vi "Heat2D_X Extend U(n).vi"(5 "Coefficients":T1={"rx"=0.0, "ry"=0.0, "s"=-0.0, "c"=0.0, "deltaT"=0.0, "deltaX"=0.0, "deltaY"=0.0}, 7 "step":i32, 10 "U(n)":dbl[][](array[numeric]), 11 "Boundary Condition":cluster{"type":T2, "Value":dbl[][]}[](array[cluster]) {"type" items=["Dirichlet", "Neumann"]}) -> (2 "Interp(X)":dbl[][](array[numeric]))   [LabVIEW 2017, in "NI_PDE.lvlib"]
uses:
  <vilib>/gmath/NI_PDE.lvlib
  <vilib>/gmath/pde.llb/Common/PDE_BC Type.ctl
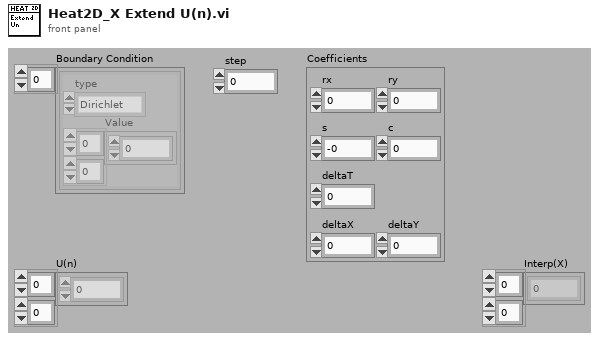
[diagram p1: front panel]
types:
  T1 = cluster{"rx":dbl, "ry":dbl, "s":dbl, "c":dbl, "deltaT":dbl, "deltaX":dbl, "deltaY":dbl}
  T2 = typedef "NI_PDE.lvlib/PDE_BC Type.ctl" = i32
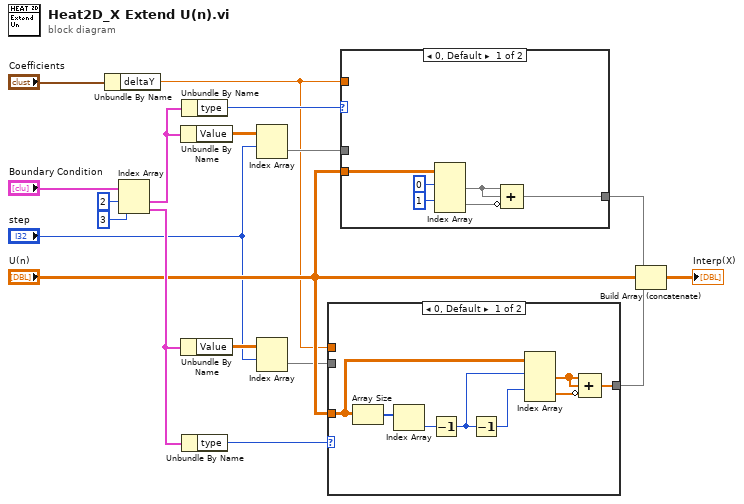
[diagram p0: block diagram]
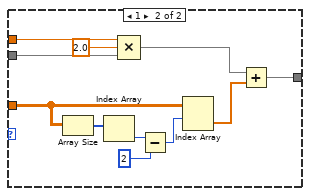
[diagram p2: hidden frame]
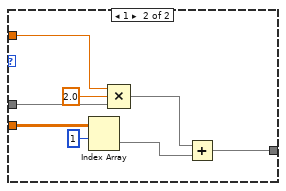
[diagram p3: hidden frame]
diagram:
  n1 = Unbundle By Name("Coefficients") -> ("deltaY"=w2:dbl)
  n2 = Index Array(array="Boundary Condition", index #1=2 ("index"), index #2=3 ("index")) -> (element #1=w11:cluster{"type":T2, "Value":dbl[][]}, element #2=w6:cluster{"type":T2, "Value":dbl[][]})
  n3 = Unbundle By Name(w11) -> ("Value"=w10:dbl[][])
  n4 = Unbundle By Name(w6) -> ("Value"=w5:dbl[][])
  n5 = Unbundle By Name(w11) -> ("type"=w12:T2)
  n6 = Unbundle By Name(w6) -> ("type"=w7:T2)
  n7 = Index Array(array=w10, index (row)="step") -> (element=w9:dbl[])  [unwired: 1 in]
  n8 = Index Array(array=w5, index (row)="step") -> (element=w3:dbl[])  [unwired: 1 in]
  n9 = case shown="0, Default" w7 {
    tunnel: [w26 w28] -> w17
    tunnel: "U(n)" -> [w19 w35]
    tunnel: w3 -> [_ w31]
    tunnel: w2 -> [_ w30]
    frame 0, Default {
      n10 = Array Size(array=w19) -> (size(s)=w25:i32[])
      n11 = Index Array(array=w25) -> (element=w24:i32)  [unwired: 1 in]
      n12 = Decrement(x=w24) -> (x-1=w20:i32)
      n13 = Decrement(x=w20) -> (x-1=w23:i32)
      n14 = Index Array(array=w19, index (row) #1=w20, index (row) #2=w23) -> (element #1=w22:dbl[], element #2=w21:dbl[])  [unwired: 2 in]
      n15 = Compound Arithmetic op=ADD(w22, w22, invert w21) -> (w26:dbl[])
    }
    frame 1 {
      n16 = Array Size(array=w35) -> (size(s)=w37:i32[])
      n17 = Index Array(array=w37) -> (element=w36:i32)  [unwired: 1 in]
      n18 = Compound Arithmetic op=MULTIPLY(w30, 2.0, w31) -> (w29:dbl[])
      n19 = Subtract(x=w36, y=2 ("index (row)")) -> (x-y=w33:i32)
      n20 = Index Array(array=w35, index (row)=w33) -> (element=w27:dbl[])  [unwired: 1 in]
      n21 = Add(x=w29, y=w27) -> (x+y=w28:dbl[])
    }
  }
  n22 = case shown="0, Default" w12 {
    tunnel: [w43 w48] -> w18
    tunnel: "U(n)" -> [w38 w51]
    tunnel: w9 -> [_ w47]
    tunnel: w2 -> [_ w46]
    frame 0, Default {
      n23 = Index Array(array=w38, index (row) #1=0 ("index (row)"), index (row) #2=1 ("index (row)")) -> (element #1=w42:dbl[], element #2=w39:dbl[])  [unwired: 2 in]
      n24 = Compound Arithmetic op=ADD(w42, w42, invert w39) -> (w43:dbl[])
    }
    frame 1 {
      n25 = Index Array(array=w51, index (row)=1) -> (element=w49:dbl[])  [unwired: 1 in]
      n26 = Compound Arithmetic op=MULTIPLY(w46, 2.0, w47) -> (w44:dbl[])
      n27 = Add(x=w44, y=w49) -> (x+y=w48:dbl[])
    }
  }
  n28 = Build Array (concatenate)(w18, "U(n)", w17) -> (→"Interp(X)":dbl[][])
